vi "Format Error String.vi"(8 "error in (no error)":errorcluster, 9 "Source":string, 10 "Code":i32) -> (0 "error out":errorcluster, 3 "Error String":string)   [LabVIEW 2020, in "Error Handler.lvlib"]
uses:
  Error Handler.lvlib
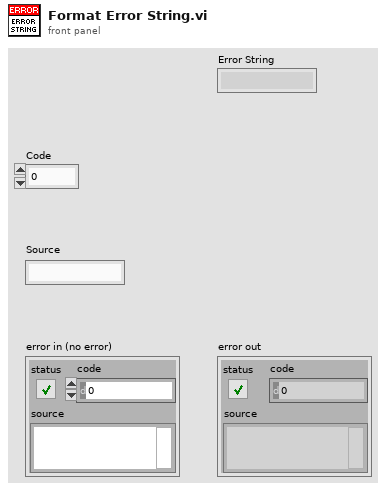
[diagram p1: front panel]
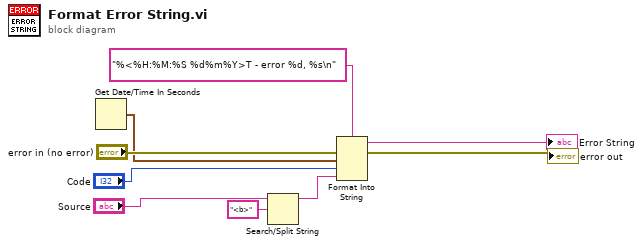
[diagram p0: block diagram]
diagram:
  n1 = Get Date/Time In Seconds() -> (seconds since 1Jan1904=w7:timestamp)
  n2 = Search/Split String(string="Source", search string/char (-)="<b>") -> (substring before match=w6:string)  [unwired: 1 in, 2 out]
  n3 = Format Into String(format string="%<%H:%M:%S %d%m%Y>T - error %d, %s\n", error in="error in (no error)", w7, "Code", w6) -> (resulting string=→"Error String":string, error out=→"error out":errorcluster)  [unwired: 1 in]
